vi "Create (robot only).vi"(6 "Worktable Mode":T1, 7 "Virtual Mode":bool, 8 "error in":errorcluster, 9 "HOME?":bool, 10 "Config Folder":path=path "C:/Users/husker/Desktop/gantry/Config") -> (0 "error out":errorcluster, 3 "Gantry out":refnum<class "Gantry Class.lvclass">)   [LabVIEW 2011, in "Gantry Class.lvclass"]
uses:
  Gantry Class.lvclass
  WorkTable Class/Type Definitions/Worktable_Mode.ctl
  Gantry Class.lvclass/Gantry Class.ctl
  Config Manager Class/Config Manager Class.lvclass
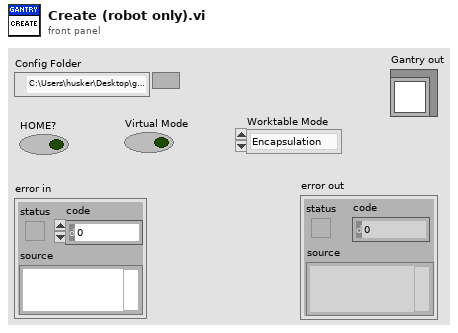
[diagram p1: front panel]
types:
  T1 = typedef "Worktable_Mode.ctl" = enum16{"Encapsulation", "Gluing"}
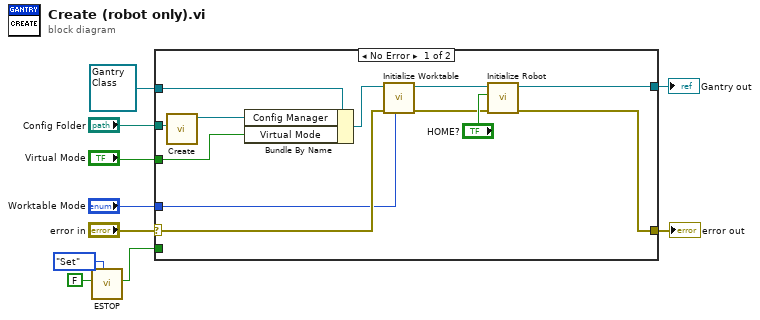
[diagram p0: block diagram]
diagram:
  n1 = call "ESTOP.vi"("Get/Set"=enum16{"Get", "Set"}."Set", "Value In"=FALSE) -> ("Value Out"=w1:bool)  [unwired: 9 in]
  n2 = case shown="No Error" "error in" {
    selector: "error in" -> [w18 w24]
    tunnel: [w11 w24] -> w9
    tunnel: [w12 w23] -> w7
    tunnel: refnum<class "Gantry Class.lvclass"> refnum ("Gantry Class in") -> [w21 w23]
    tunnel: "Config Folder" -> [w20 _]
    tunnel: "Virtual Mode" -> [w22 _]
    tunnel: "Worktable Mode" -> [w15 _]
    tunnel: w1 -> [_ _]
    frame No Error {
      n3 = call "Create.vi"("Config Files Directory"=w20) -> ("Config Manager out"=w19:refnum<class "Config Manager Class.lvclass">)  [unwired: 9 in, 1 out]
      n4 = Bundle By Name(cluster=w21, "Config Manager"=w19, "Virtual Mode"=w22) -> (w17:refnum<class "Gantry Class.lvclass">)
      n5 = call-dynamic "Initialize Worktable.vi"("Worktable Mode"=w15, "error in"=w18, "Gantry in"=w17) -> ("error out"=w13:errorcluster, "Gantry out"=w14:refnum<class "Gantry Class.lvclass">)  [unwired: 7 in]
      n6 = call-dynamic "Initialize Robot.vi"("error in"=w13, "HOME?"="HOME?", "Gantry in"=w14) -> ("error out"=w11:errorcluster, "Gantry out"=w12:refnum<class "Gantry Class.lvclass">)  [unwired: 7 in]
    }
    frame Error {
    }
  }
  "error out" <- w9
  "Gantry out" <- w7
